vi "Setup.vi"(8 "error in (no error)":errorcluster, 11 "LUnit Test FInder Test In":refnum<class "Test FInder Test.lvclass">) -> (0 "error out":errorcluster, 3 "LUnit Test FInder Test Out":refnum<class "Test FInder Test.lvclass">)   [LabVIEW 2020, in "Test FInder Test.lvclass"]
doc: "Setup method called by the testing framework before each test method is called."
uses:
  Test FInder Test.lvclass
  source/User Interface/Support/Utilities.lvlib
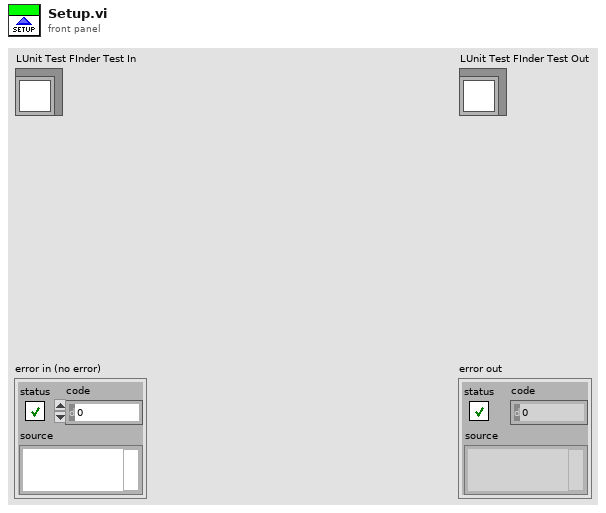
[diagram p1: front panel]
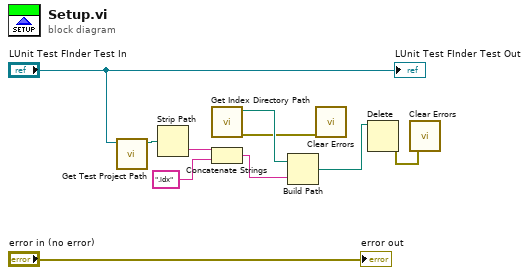
[diagram p0: block diagram]
diagram:
  n1 = call "Get Test Project Path.vi"("LUnit Test Suite Tests in"="LUnit Test FInder Test In") -> ("appended path"=w1:path)  [unwired: 10 in]
  n2 = Strip Path(path=w1) -> (name=w5:string)  [unwired: 1 out]
  n3 = call "Get Index Directory Path.vi"() -> ("error out"=w4:errorcluster, "Index Directory"=w7:path)  [unwired: 10 in]
  n4 = Concatenate Strings(w5, ".idx" ("string")) -> (w8:string)
  n5 = Build Path(base path=w7, name or relative path=w8) -> (appended path=w3:path)
  n6 = call <vilib>:"Clear Errors.vi"("error in (no error)"=w4) -> ()  [unwired: 5 in, 2 out]
  n7 = Delete(path (use dialog)=w3) -> (error out=w9:errorcluster)  [unwired: 4 in, 2 out]
  n8 = call <vilib>:"Clear Errors.vi"("error in (no error)"=w9) -> ()  [unwired: 5 in, 2 out]
  "error out" <- "error in (no error)"
  "LUnit Test FInder Test Out" <- "LUnit Test FInder Test In"
